vi "Read Registers.vi"(8 "error in (no error)":errorcluster, 11 "Serial Config":T2={"串口选择"="", "通讯速率"=9600, "超时时间"=200, "数据位长"=8, "奇偶校验"=enum."None", "停止位长"=10, "握手控制"=0, "字符结束"=TRUE, "结束字符"=10, "仪器地址"=1} {"结束字符" format="%.0x"; "握手控制" items=["None", "XON/XOFF", "RTS/CTS", "XON/XOFF & RTS/CTS", "DTR/DSR", "XON/XOFF & DTR/DSR"]; "停止位长" items=["1.0"=10, "1.5"=15, "2.0"=20]; "数据位长" min=5 max=8 step=1}) -> (0 "error out":errorcluster, 2 "Status Code":string, 3 "Registers":T1)   [LabVIEW 2010, in "DCP551.lvlib"]
uses:
  DCP551.lvlib
  <vilib>/Instr/_visa.llb/VISA Configure Serial Port (Instr).vi
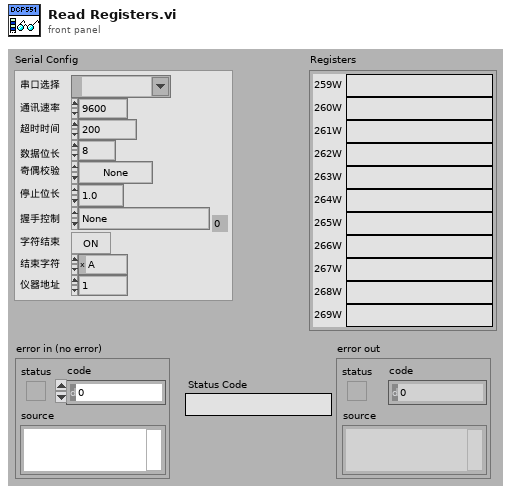
[diagram p1: front panel]
types:
  T1 = cluster{"259W":string, "260W":string, "261W":string, "262W":string, "263W":string, "264W":string, "265W":string, "266W":string, "267W":string, "268W":string, "269W":string}
  T2 = cluster{"串口选择":refnum<visa-resource-name>, "通讯速率":u32, "超时时间":u32, "数据位长":u16, "奇偶校验":enum16{"None", "Odd", "Even", "Mark", "Space"}, "停止位长":u16, "握手控制":u16, "字符结束":bool, "结束字符":u8, "仪器地址":u32}
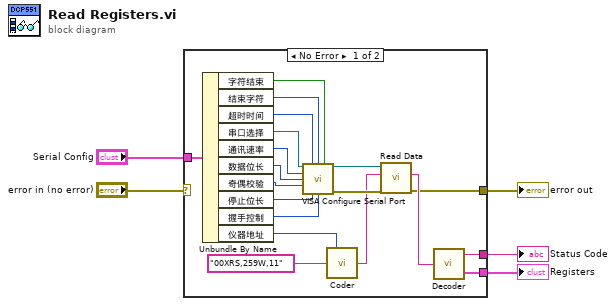
[diagram p0: block diagram]
diagram:
  n1 = case shown="No Error" "error in (no error)" {
    selector: "error in (no error)" -> [_ w25]
    tunnel: "Serial Config" -> [w15 _]
    tunnel: [w10 w25] -> w3
    tunnel: [w9 _] -> w2
    tunnel: [w8 _] -> w1
    frame No Error {
      n2 = Unbundle By Name(w15) -> ("字符结束"=w18:bool, "结束字符"=w17:u8, "超时时间"=w16:u32, "串口选择"=w24:refnum<visa-resource-name>, "通讯速率"=w23:u32, "数据位长"=w22:u16, "奇偶校验"=w21:enum16{"None", "Odd", "Even", "Mark", "Space"}, "停止位长"=w20:u16, "握手控制"=w19:u16, "仪器地址"=w7:u32)
      n3 = call-poly "VISA Configure Serial Port"("VISA resource name"=w24, "timeout (10sec)"=w16, "termination char\n(0xA = '\\n' = LF)"=w17, "Enable Termination\nChar (T)"=w18, "baud rate (9600)"=w23, "data bits (8)"=w22, "parity (0:none)"=w21, "stop bits (10: 1 bit)"=w20, "flow control (0:none)"=w19) -> ("VISA resource name out"=w14:refnum<visa-resource-name>, "error out"=w13:errorcluster)  [unwired: 1 in, 4 out]
      n4 = call "Coder.vi"("Station Address"=w7, "Input"="00XRS,259W,11" ("string")) -> ("Output"=w12:string)  [unwired: 13 in]
      n5 = call "Read Data.vi"("error in (no error)"=w13, "COMMAND"=w12, "VISA resource name in"=w14) -> ("error out"=w10:errorcluster, "Output"=w11:string)  [unwired: 6 in, 1 out]
      n6 = call "Decoder.vi"("Input"=w11) -> ("Registers"=w8:T1, "Status Code"=w9:string)
    }
    frame Error {
    }
  }
  "error out" <- w3
  "Status Code" <- w2
  "Registers" <- w1
